vi "80测试.vi"() -> ()   [LabVIEW 2018]
uses:
  <vilib>/addons/database/Connection.llb/DB Tools Open Connec (String).vi
  <vilib>/addons/database/NI_Database_API.lvlib
panel:
  in  "确定按钮":bool
  out "error out":errorcluster
  out "80二维码":string
  out "上一站号 (80)":string
  out "上一站结果 (80)":string
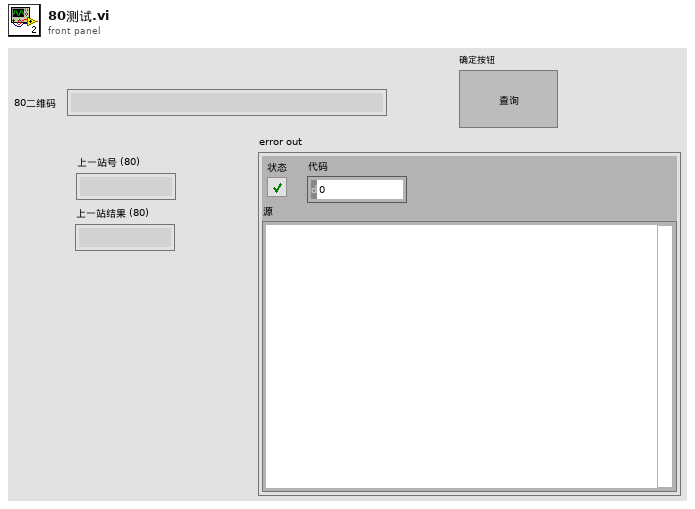
[diagram p1: front panel]
types:
  T1 = typedef "NI_Database_API.lvlib/Conn ObjectReference.ctl" = refnum<k1>
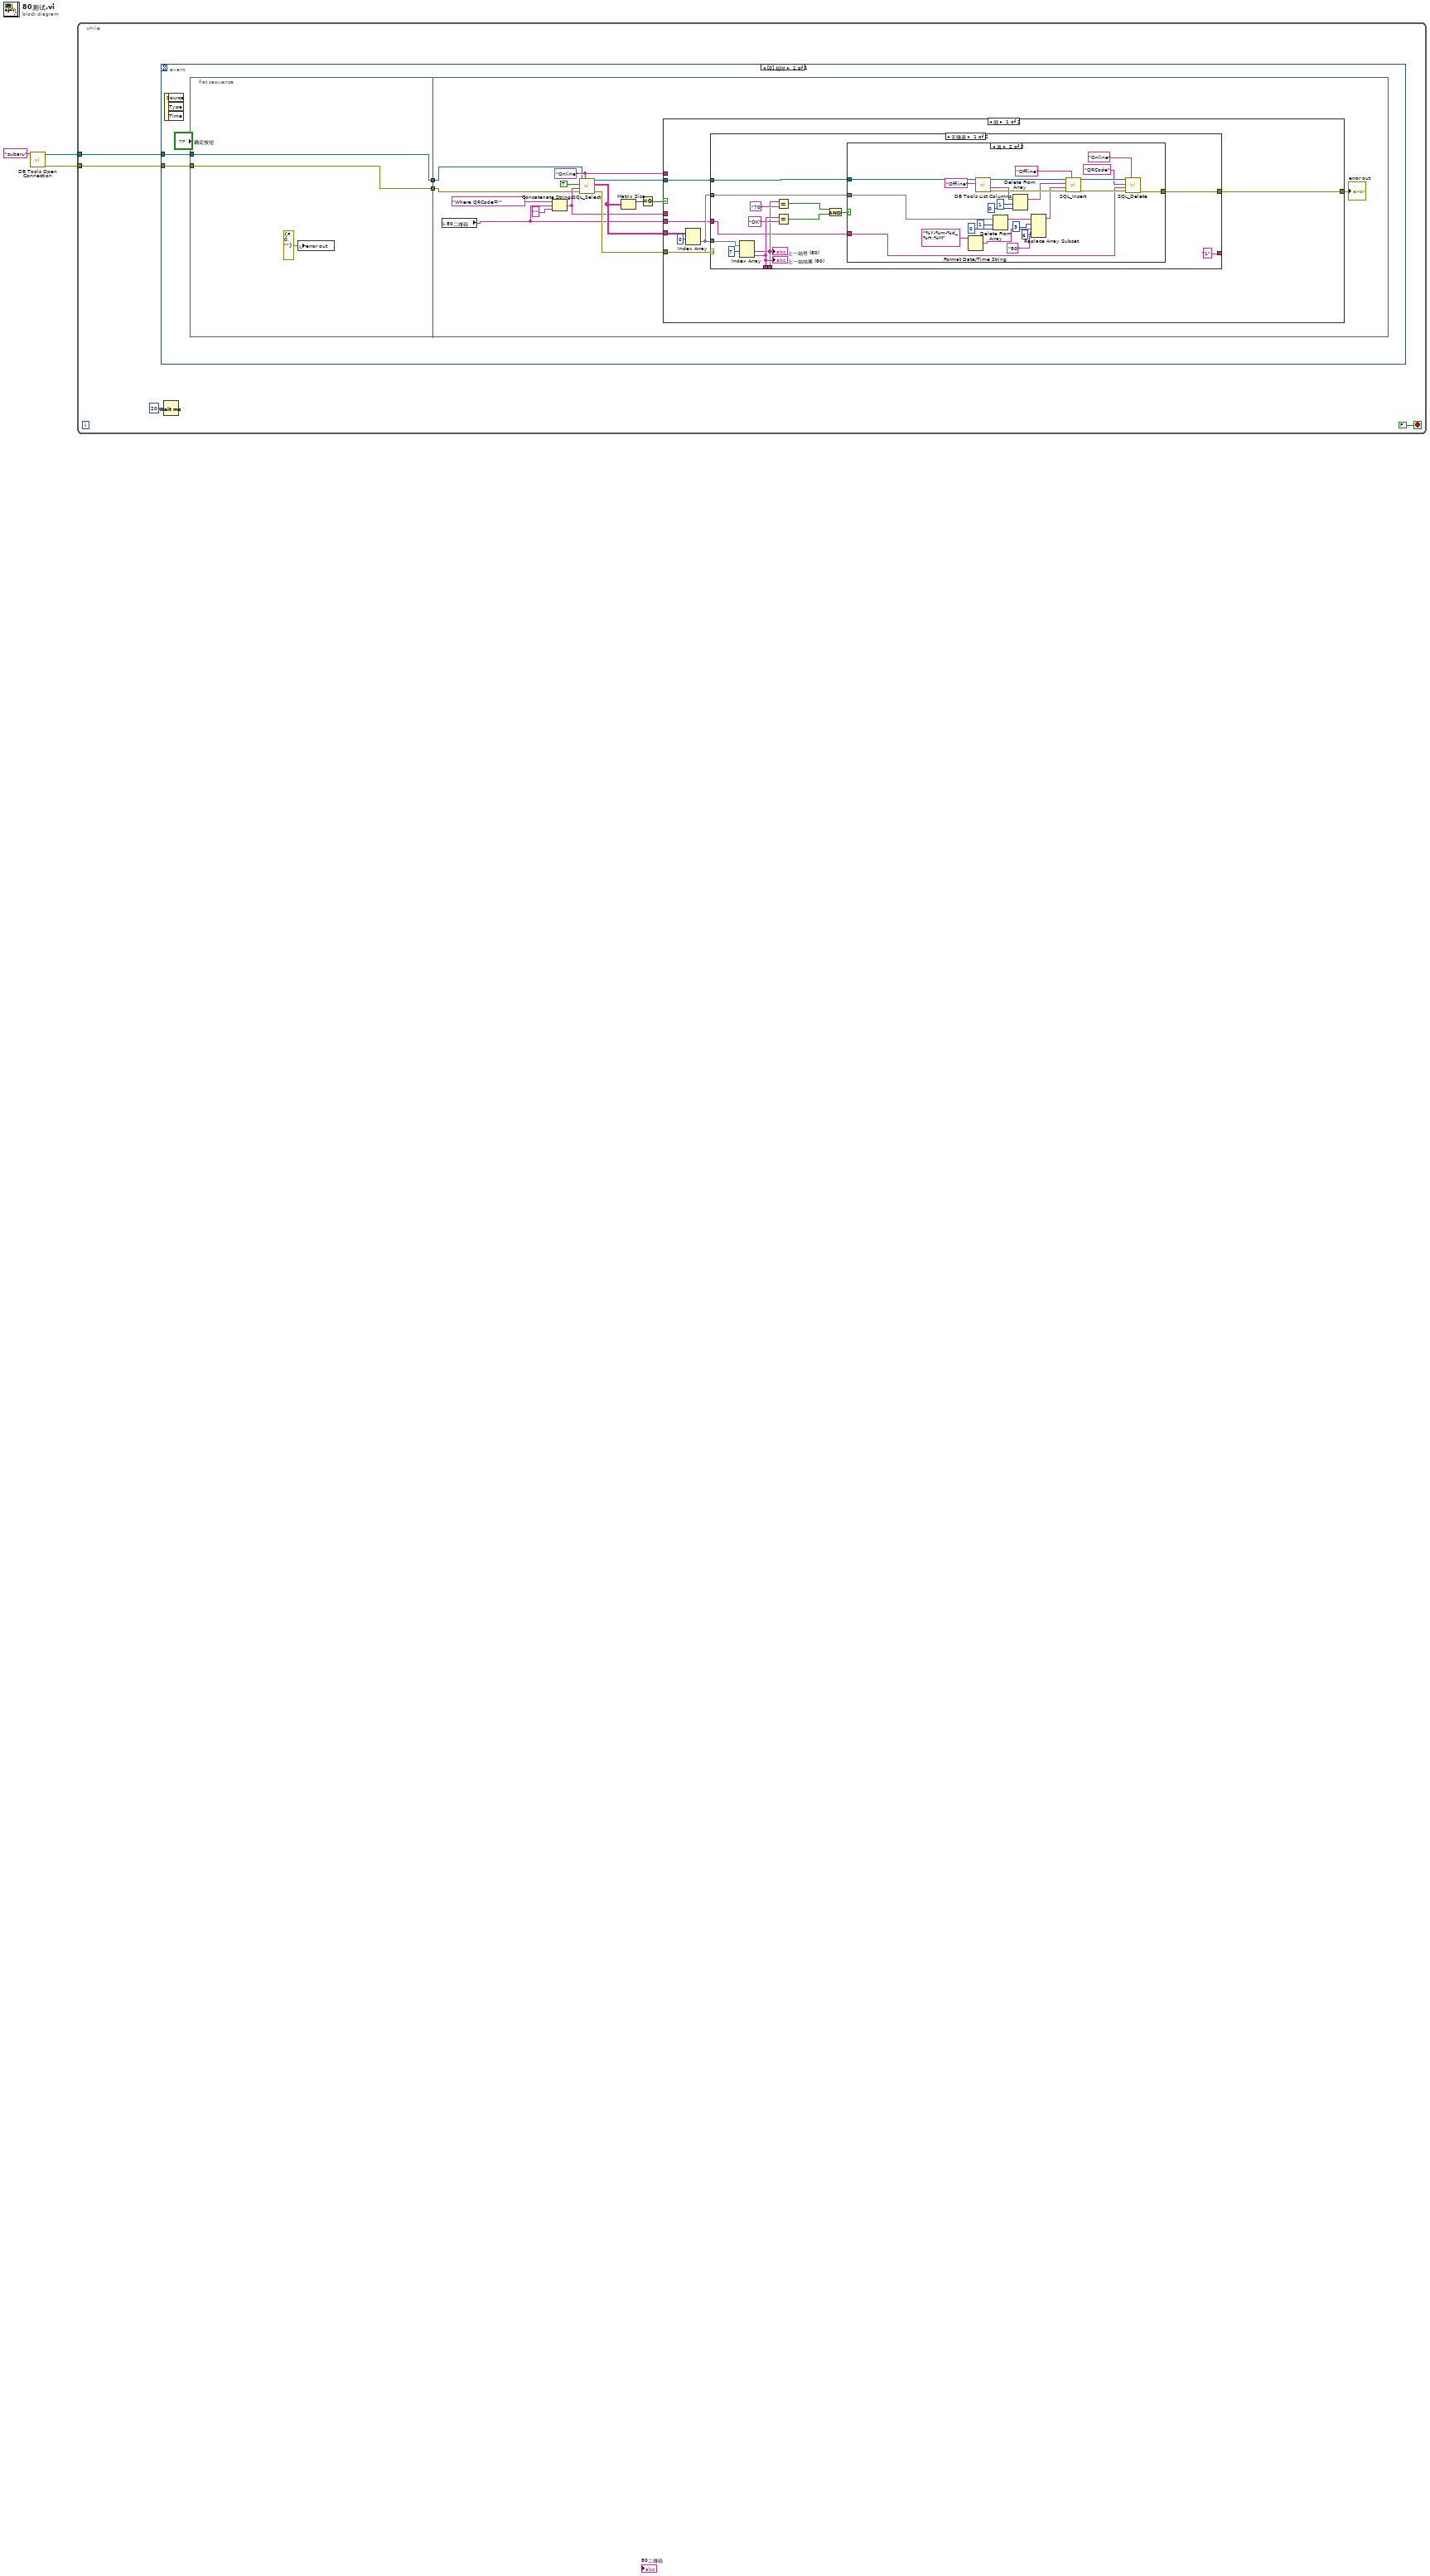
[diagram p0: block diagram]
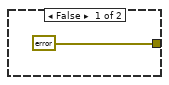
[diagram p2: hidden frame]
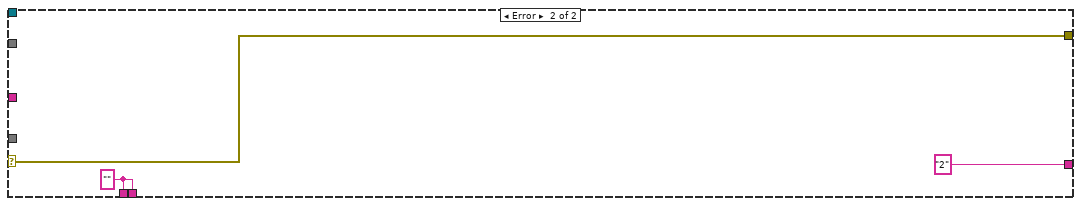
[diagram p3: hidden frame]
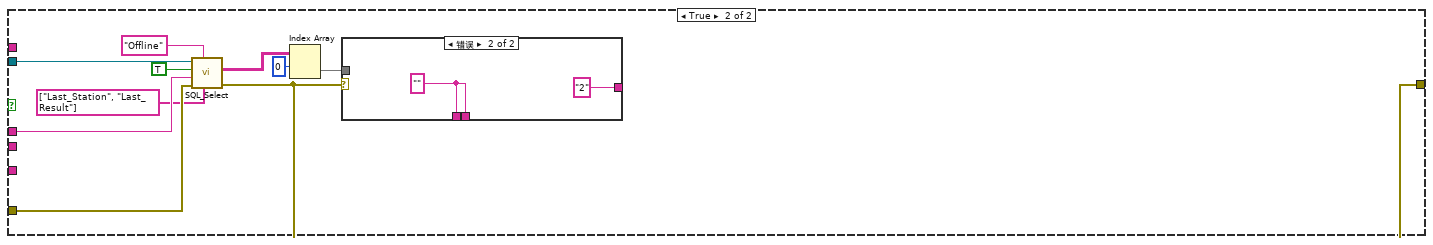
[diagram p4: hidden frame]
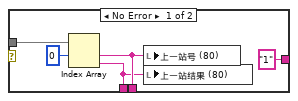
[diagram p5: hidden frame]
diagram:
  n1 = call-poly <vilib>:"DB Tools Open Connection.vi"("connection information"="subaru") -> ("error out"=w2:errorcluster, "connection reference"=w1:T1)  [unwired: 7 in]
  n2 = while {
    tunnel: w2 -> [w5]
    tunnel: w1 -> [w4]
    stop <- FALSE stop-if-true
    n3 = event shown="[0] 超时" {
      selector: _ -> [_]
      dyn-events: _ -> [_]
      timeout: _ -> [_]
      tunnel: w5 -> [w9]
      tunnel: w4 -> [w8]
      event Timeout {
        n4 = event-data() -> ()  [unwired: 1 in, 3 out]
        n5 = flat-sequence {
          tunnel: [w12] -> w11
          tunnel: [w13] -> w10
          tunnel: w9 -> [w13]
          tunnel: w8 -> [w12]
          tunnel: w11 -> [w16]
          tunnel: w10 -> [w15]
          frame #0 {
            n6 = local write "error out"(errorcluster {"status"=FALSE, "code"=0, "source"=""} ("error out")) -> ()
          }
          frame #1 {
            w23 = "Online" ("表名")
            n7 = local read "80二维码"() -> (w18:string)
            n8 = Concatenate Strings("Where QRCode='" ("查询语句"), w18, "'" ("字符串")) -> (w19:string)
            n9 = call "SQL_Select.vi"("表名"=w23, "error in (no error)"=w15, "查询语句"=w19, "查询条件"=TRUE, "connection reference"=w16) -> ("error out"=w25:errorcluster, "数据"=w26:string[][], "connection reference out"=w24:T1)  [unwired: 4 in]
            n10 = Matrix Size(0:w26) -> (1:w27:i32)  [unwired: 1 out]
            n11 = Equal To 0?(x=w27) -> (x = 0?=w28:bool)
            n12 = case shown="假" w28 {
              tunnel: w25 -> [w35 w85]
              tunnel: w24 -> [w32 w87]
              tunnel: w23 -> [_ _]
              tunnel: w26 -> [w33 _]
              tunnel: w18 -> [w30 _]
              tunnel: [w29 w81] -> w17
              tunnel: w19 -> [_ w86]
              frame False {
                n13 = Index Array(array=w33, index (row)=0 ("索引 (行)")) -> (element=w31:string[])  [unwired: 1 in]
                n14 = case shown="无错误" w35 {
                  selector: w35 -> [_ w76]
                  tunnel: ["1" ("右扫码请求回复") "2" ("右扫码请求回复")] -> _
                  tunnel: [w38 w77] -> _
                  tunnel: [w45 w77] -> _
                  tunnel: w31 -> [w47 _]
                  tunnel: w32 -> [w41 _]
                  tunnel: w31 -> [w40 _]
                  tunnel: w30 -> [w36 _]
                  tunnel: [w39 w76] -> w29
                  frame No Error {
                    n15 = Index Array(array=w47, index #1=7 ("索引 (行)")) -> (element #1=w38:string, element #2=w45:string)  [unwired: 1 in]
                    "上一站号 (80)" <- w38
                    "上一站结果 (80)" <- w45
                    n16 = Equal?(x=w38, y="70") -> (x = y?=w37:bool)
                    n17 = Equal?(x=w45, y="OK") -> (x = y?=w43:bool)
                    n18 = And(x=w37, y=w43) -> (x .and. y?=w42:bool)
                    n19 = case shown="真" w42 {
                      tunnel: w41 -> [_ w56]
                      tunnel: w40 -> [_ w55]
                      tunnel: w36 -> [_ w53]
                      tunnel: [errorcluster {"status"=FALSE, "code"=0, "source"=""} ("error out") w54] -> w39
                      frame False {
                      }
                      frame True {
                        n20 = Format Date/Time String(time format string (%c)="%Y-%m-%d_%H:%M" ("时间格式字符串(%c)")) -> (date/time string=w68:string)  [unwired: 2 in]
                        n21 = call <vilib>:"DB Tools List Columns.vi"("table"="Offline" ("表名"), "connection reference"=w56) -> ("error out"=w73:errorcluster, "columns"=w74:string[], "connection reference out"=w75:T1)  [unwired: 2 in, 1 out]
                        n22 = Delete From Array(array=w55, length=1 ("长度"), index=0 ("索引")) -> (array with subset deleted=w69:string[])  [unwired: 1 out]
                        n23 = Delete From Array(array=w74, length=1 ("长度"), index=0 ("索引")) -> (array with subset deleted=w72:string[])  [unwired: 1 out]
                        n24 = Replace Array Subset(array=w69, new element #1=w68, index #1=3 ("索引"), new element #2="80" ("新元素/子数组"), index #2=6 ("索引")) -> (w67:string[])
                        n25 = call "SQL_Insert.vi"("表名"="Offline", "error in (no error)"=w73, "值"=w67, "列名"=w72, "connection reference"=w75) -> ("error out"=w70:errorcluster, "connection reference 2"=w71:T1)  [unwired: 5 in]
                        n26 = call "SQL_Delete.vi"("表名"="Online", "error in (no error)"=w70, "值"=w53, "列名"="QRCode", "connection reference"=w71) -> ("error out"=w54:errorcluster)  [unwired: 5 in, 1 out]
                      }
                    }
                  }
                  frame Error {
                    w77 = ""
                  }
                }
              }
              frame True {
                n27 = call "SQL_Select.vi"("要读取的列名"=string[] ["Last_Station", "Last_Result"], "表名"="Offline", "error in (no error)"=w85, "查询语句"=w86, "查询条件"=TRUE, "connection reference"=w87) -> ("error out"=w81:errorcluster, "数据"=w82:string[][])  [unwired: 3 in, 1 out]
                n28 = Index Array(array=w82, index (row)=0 ("索引 (行)")) -> (element=w83:string[])  [unwired: 1 in]
                n29 = case shown="错误" w81 {
                  tunnel: ["1" ("右扫码请求回复") "2" ("右扫码请求回复")] -> _
                  tunnel: [w90 w94] -> _
                  tunnel: [w89 w94] -> _
                  tunnel: w83 -> [w91 _]
                  frame No Error {
                    n30 = Index Array(array=w91, index #1=0 ("索引 (行)")) -> (element #1=w90:string, element #2=w89:string)  [unwired: 1 in]
                    n31 = local write "上一站号 (80)"(w90) -> ()
                    n32 = local write "上一站结果 (80)"(w89) -> ()
                  }
                  frame Error {
                    w94 = ""
                  }
                }
              }
            }
            "error out" <- w17
          }
        }
      }
    }
    n33 = Wait (ms)(milliseconds to wait=u32 20 ("等待时间（毫秒）")) -> ()  [unwired: 1 out]
  }
